vi "写入指令事件.vi"(8 "error in (no error)":errorcluster caption="错误输入（无错误）", 10 "指令事件":refnum<user-event>, 11 "客户端输入":refnum<class "客户端.lvclass">) -> (0 "error out":errorcluster caption="错误输出", 3 "客户端输出":refnum<class "客户端.lvclass">)   [LabVIEW 2015, in "客户端操作者.lvlib" / "客户端.lvclass"]
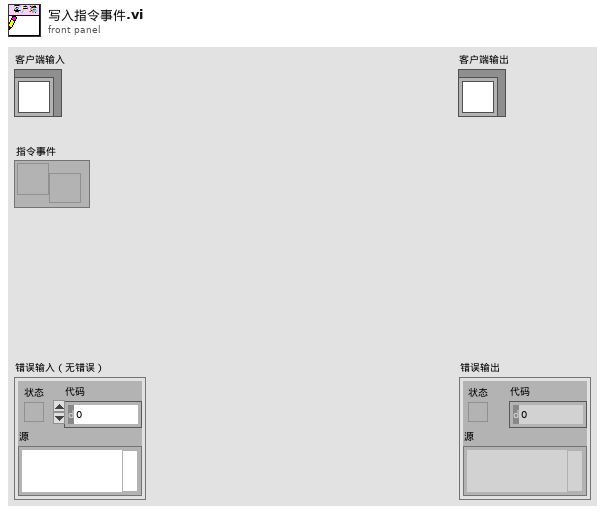
[diagram p1: front panel]
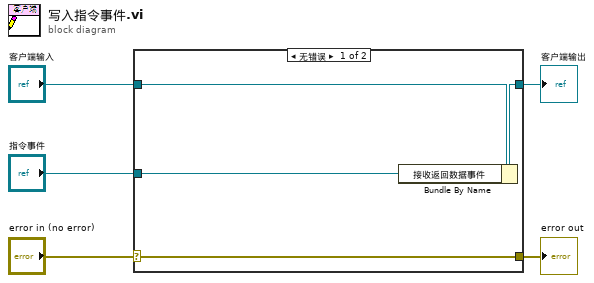
[diagram p0: block diagram]
diagram:
  n1 = case shown="无错误" "error in (no error)" {
    selector: "error in (no error)" -> [w9 w10]
    tunnel: [w9 w10] -> w4
    tunnel: [w7 w11] -> w2
    tunnel: "客户端输入" -> [w8 w11]
    tunnel: "指令事件" -> [w6 _]
    frame No Error {
      n2 = Bundle By Name(cluster=w8, "接收返回数据事件"=w6) -> (w7:refnum<class "客户端.lvclass">)
    }
    frame Error {
    }
  }
  "error out" <- w4
  "客户端输出" <- w2
